vi "Auto Match.vi"() -> ()   [LabVIEW 2015]
panel:
  out "Number of Iterations":i32
  out "Current Number":dbl
  in  "Number to Match":dbl=50.0 max=1000.0 step=1.0
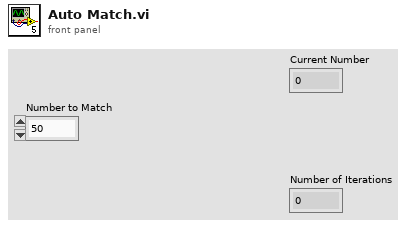
[diagram p1: front panel]
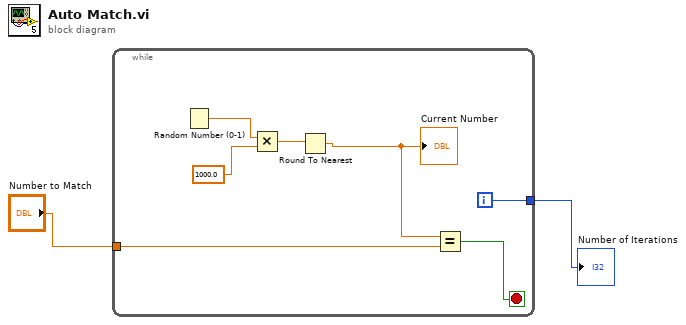
[diagram p0: block diagram]
diagram:
  n1 = while {
    tunnel: "Number to Match" -> [w6]
    tunnel: [w3] -> w1
    i -> [w3]
    stop <- w4 stop-if-true
    n2 = Random Number (0-1)() -> (number: 0 to 1=w9:dbl)
    n3 = Multiply(x=w9, y=1000.0) -> (x*y=w7:dbl)
    n4 = Round To Nearest(number=w7) -> (nearest integer value=w5:dbl)
    "Current Number" <- w5
    n5 = Equal?(x=w5, y=w6) -> (x = y?=w4:bool)
  }
  "Number of Iterations" <- w1
